vi "Check If point on Line.vi"(8 "Error In":errorcluster, 9 "Original Bearing":dbl, 10 "Point in question":T1 {"Latitude" format="%#_10g"; "Longitude" format="%#_10g"}, 11 "Origin Point":T1 {"Latitude" format="%#_10g"; "Longitude" format="%#_10g"}) -> (0 "Error Out":errorcluster, 3 "In Range?":bool)   [LabVIEW 2014]
uses:
  Lat Long Conversion/Controls/PointLatLon.ctl
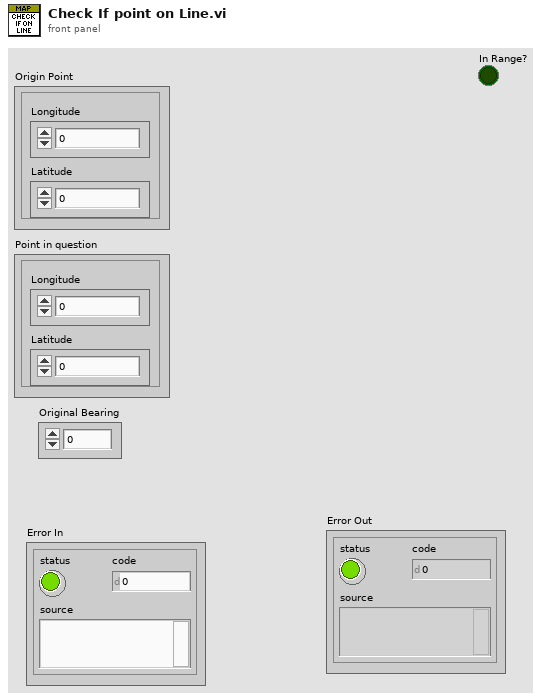
[diagram p1: front panel]
types:
  T1 = typedef "PointLatLon.ctl" = cluster{"Longitude":dbl, "Latitude":dbl}
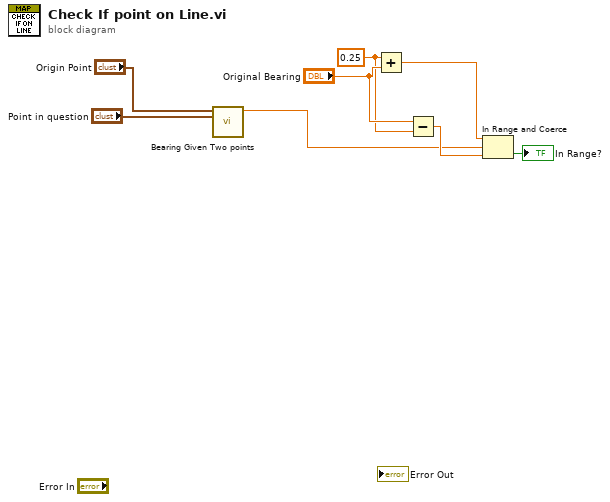
[diagram p0: block diagram]
diagram:
  w5 = 0.25 ("x")
  n1 = call "Bearing Given Two points.vi"("End Point"="Point in question", "Origin Point"="Origin Point") -> ("Bearing (True North)"=w2:dbl)  [unwired: 8 in, 1 out]
  n2 = Add(x=w5, y="Original Bearing") -> (x+y=w4:dbl)
  n3 = Subtract(x="Original Bearing", y=w5) -> (x-y=w3:dbl)
  n4 = In Range and Coerce(upper limit=w4, x=w2, lower limit=w3) -> (In Range?=→"In Range?":bool)  [unwired: 1 out]
